vi "FTW-ActorContext-Destroy.vi"(0 "Actor Context":refnum<class "FTW-Actor-Context.lvclass">, 11 "error in":errorcluster) -> (15 "error out":errorcluster)   [LabVIEW 2015, in "FTW-Actor-Context.lvclass"]
uses:
  FTW-Actor-Context.lvclass
  FTW-Actor-Context.lvclass/FTW-Actor-Context.ctl
panel:
  # "Inputs"
  # "Outputs"
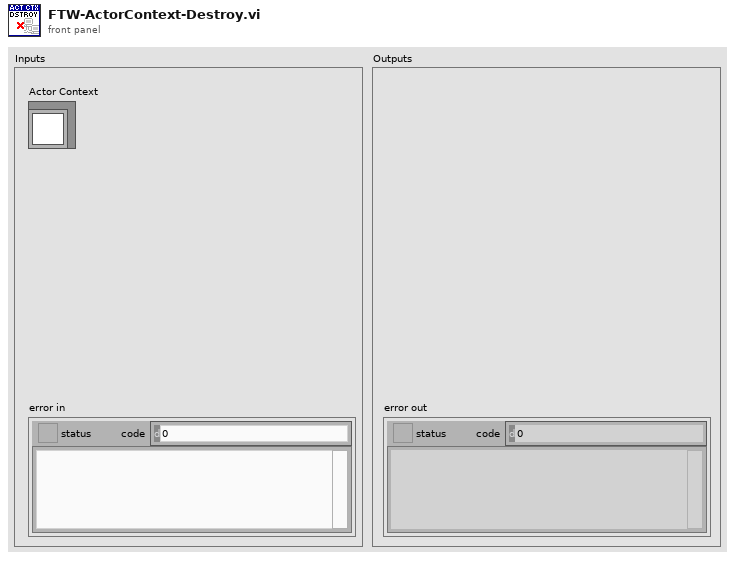
[diagram p1: front panel]
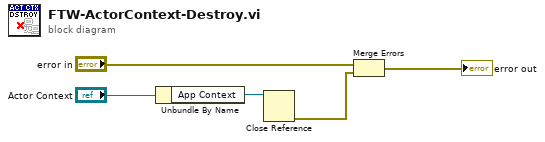
[diagram p0: block diagram]
diagram:
  n1 = Unbundle By Name("Actor Context") -> ("App Context"=w4:refnum<vi>)
  n2 = Close Reference(reference=w4) -> (error out=w1:errorcluster)  [unwired: 1 in]
  n3 = Merge Errors("error in", w1) -> (→"error out":errorcluster)
